vi "Pulse.vi"(10 "Input":bool, 11 "Rising Edge?":bool=TRUE) -> (2 "Output":bool)   [LabVIEW 2016]
panel:
  # "Sends out  a pulse only on the iteration the Input changes from false to true."
  # "Could be used when you want a joystick action to only happen once."
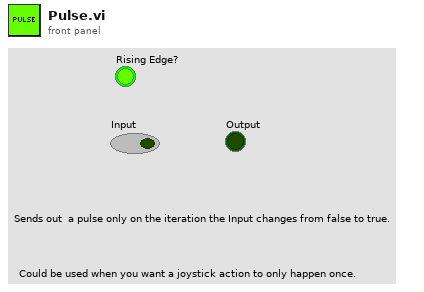
[diagram p1: front panel]
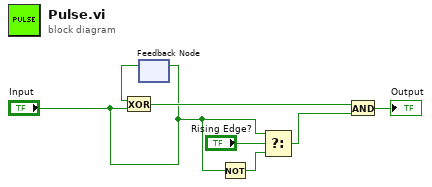
[diagram p0: block diagram]
diagram:
  n1 = feedback-in #1("Input") -> ()
  n2 = feedback #1() -> (w7:bool)  [unwired: 1 in]
  n3 = Exclusive Or(1:"Input", 2:w7) -> (0:w5:bool)
  n4 = Not(x="Input") -> (.not. x?=w3:bool)
  n5 = Select(t="Input", s="Rising Edge?", f=w3) -> (s? t:f=w4:bool)
  n6 = And(x=w5, y=w4) -> (x .and. y?=→"Output":bool)
